vi "Add User.vi"(8 "error in":errorcluster, 9 "Path":path) -> (0 "error out":errorcluster)   [LabVIEW 2015]
uses:
  <vilib>/Utility/file.llb/Read Delimited Spreadsheet (string).vi
  <vilib>/Utility/file.llb/Write Delimited Spreadsheet (string).vi
panel:
  in  "hide(F)/show(T)":bool
  in  "Cancel":bool
  in  "OK":bool
  in  "User Name":string
  in  "Password":string
  in  "Designation":u16(ring) items=["Select the Designation", "Operator", "Supevisor", "Admin"]
  # "Add User Credential"
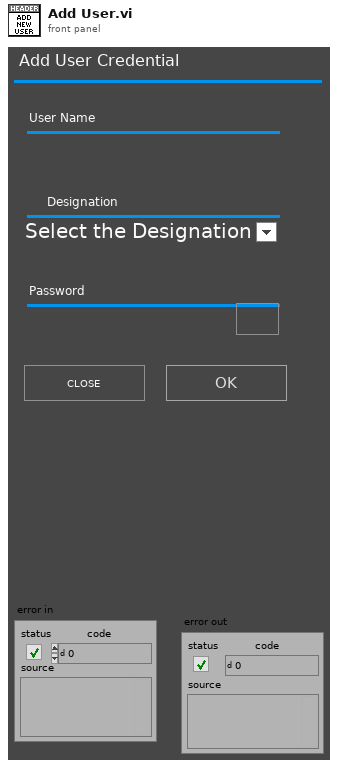
[diagram p1: front panel]
types:
  T1 = enum8{"Enabled", "Disabled", "Disabled and Grayed Out"}
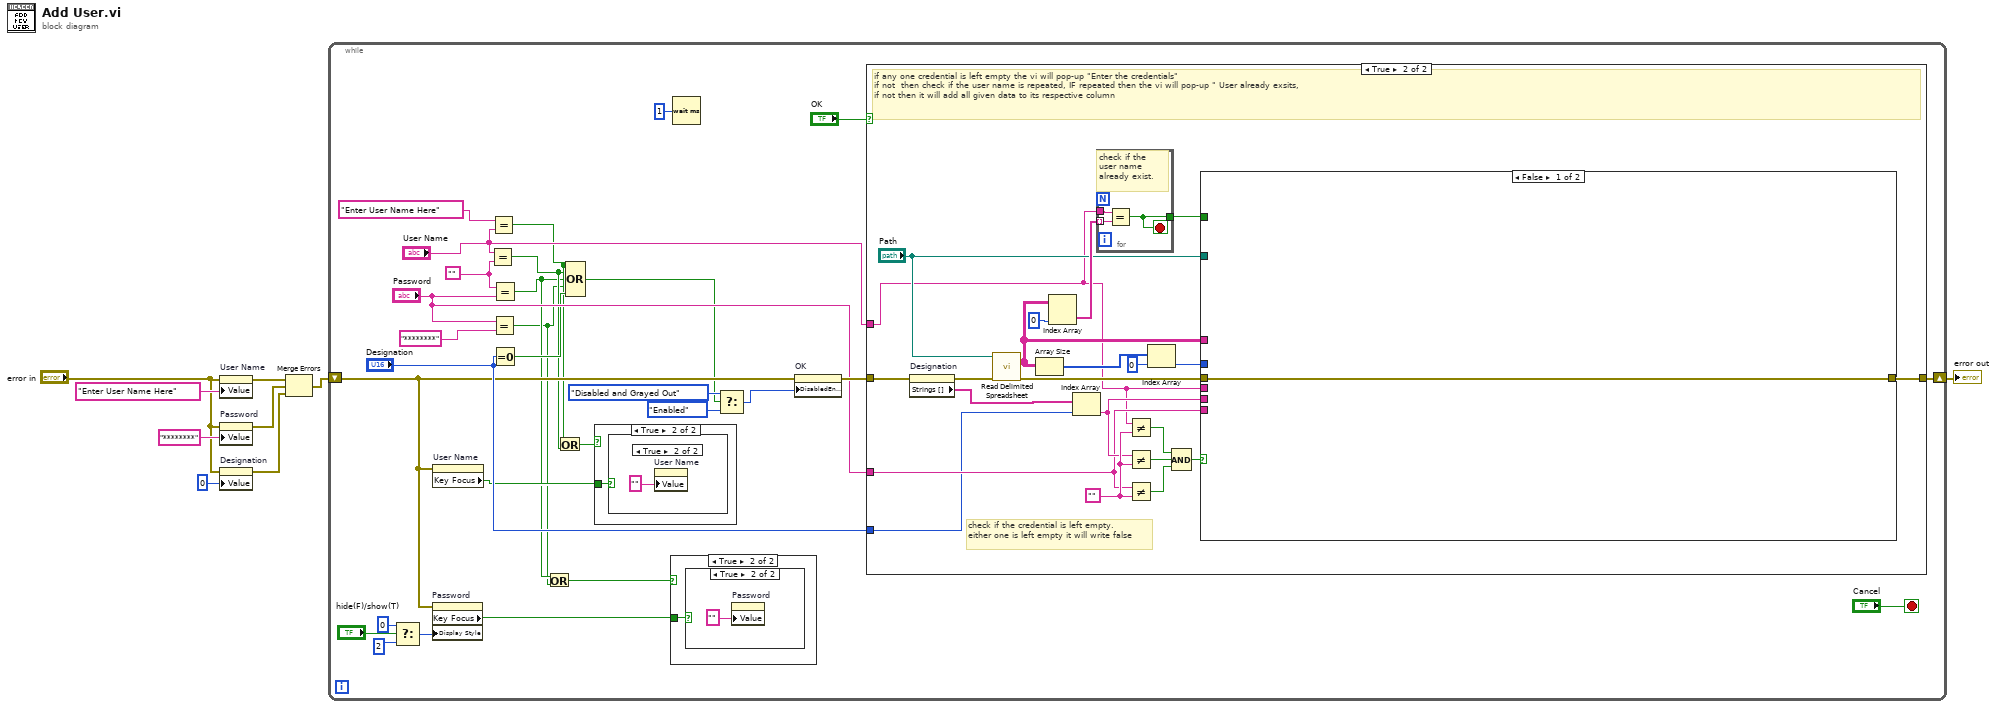
[diagram p0: block diagram]
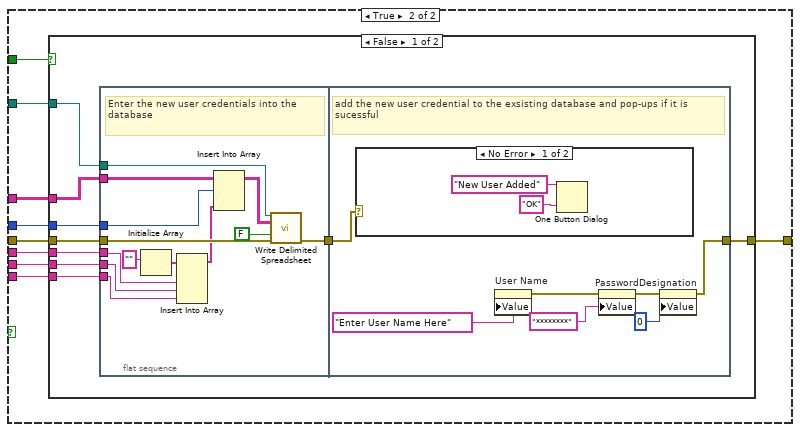
[diagram p7: hidden frame]
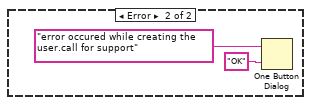
[diagram p8: hidden frame]
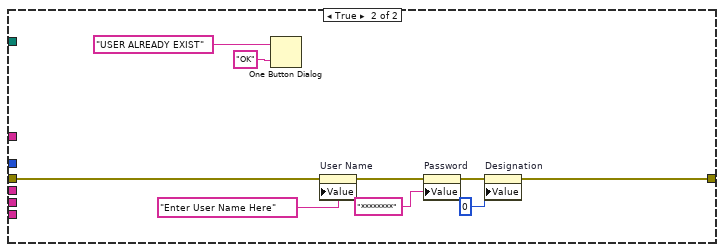
[diagram p9: hidden frame]
diagram:
  n1 = property on="User Name" class="Str"(error in="error in", "Value"="Enter User Name Here") -> (error out=w3:errorcluster)  [unwired: 1 in, 1 out]
  n2 = property on="Password" class="Str"(error in="error in", "Value"="********") -> (error out=w4:errorcluster)  [unwired: 1 in, 1 out]
  n3 = property on="Designation" class="Ring (strict)"(error in="error in", "Value"=0) -> (error out=w5:errorcluster)  [unwired: 1 in, 1 out]
  n4 = Merge Errors(w3, w4, w5) -> (w1:errorcluster)
  n5 = while {
    shift-right: [w36] -> w9
    shift-left: w1 -> [w24]
    stop <- "Cancel" stop-if-true
    w34 = ""
    n6 = Select(t=u32 0, s="hide(F)/show(T)", f=u32 2 ("Display Style")) -> (s? t:f=w11:u32)
    n7 = property on="Password" class="Str"(error in=w24, "Display Style"=w11) -> ("Key Focus"=w12:bool)  [unwired: 1 in, 2 out]
    n8 = property on="User Name" class="Str"(error in=w24) -> ("Key Focus"=w16:bool)  [unwired: 1 in, 2 out]
    n9 = Equal?(x="User Name", y=w34) -> (x = y?=w18:bool)
    n10 = Equal?(x="Enter User Name Here", y="User Name") -> (x = y?=w19:bool)
    n11 = Equal?(x="Password", y="********") -> (x = y?=w13:bool)
    n12 = Equal?(x=w34, y="Password") -> (x = y?=w14:bool)
    n13 = Equal To 0?(x="Designation") -> (x = 0?=w28:bool)
    n14 = Or(x=w14, y=w13) -> (x .or. y?=w15:bool)
    n15 = Or(x=w19, y=w18) -> (x .or. y?=w17:bool)
    n16 = Compound Arithmetic op=OR(w19, w18, w14, w13, w28) -> (w22:bool)
    n17 = case shown="True" w17 {
      tunnel: w16 -> [_ w41]
      frame False {
      }
      frame True {
        n18 = case shown="True" w41 {
          frame False {
          }
          frame True {
            n19 = property on="User Name" class="Str"("Value"="" ("User Name")) -> ()  [unwired: 2 in, 2 out]
          }
        }
      }
    }
    n20 = case shown="True" w15 {
      tunnel: w12 -> [_ w39]
      frame False {
      }
      frame True {
        n21 = case shown="True" w39 {
          frame False {
          }
          frame True {
            n22 = property on="Password" class="Str"("Value"="" ("User Name")) -> ()  [unwired: 2 in, 2 out]
          }
        }
      }
    }
    n23 = Wait (ms)(milliseconds to wait=u32 1) -> ()  [unwired: 1 out]
    n24 = Select(t=T1."Disabled and Grayed Out" ("Disabled"), s=w22, f=T1."Enabled") -> (s? t:f=w20:T1)
    n25 = property on="OK" class="Bool"(error in=w24, "DisabledEnum"=w20) -> (error out=w35:errorcluster)  [unwired: 1 in, 1 out]
    n26 = case shown="True" "OK" {
      tunnel: w35 -> [w43 w46]
      tunnel: [w43 w50] -> w36
      tunnel: "User Name" -> [_ w48]
      tunnel: "Password" -> [_ w49]
      tunnel: "Designation" -> [_ w47]
      frame False {
      }
      frame True {
        w63 = ""
        # "check if the credential is left empty. either one is left empty it will write false"
        # "if any one credential is left empty the vi will pop-up \"Enter the credentials\" \nif not  then check if the user name is repeated, IF repeated then the vi will pop-up \" User already exsits,\nif not then it will add all given data to its respective column"
        n27 = property on="Designation" class="Ring (strict)"(error in=w46) -> (error out=w45:errorcluster, "Strings []"=w44:string[])  [unwired: 1 in, 1 out]
        n28 = call-poly <vilib>:"Read Delimited Spreadsheet.vi"("file path (dialog if empty)"="Path", "error in (no error)"=w45) -> ("all rows"=w52:string[][], "error out"=w51:errorcluster)  [unwired: 8 in, 4 out]
        n29 = Array Size(array=w52) -> (size(s)=w65:i32[])
        n30 = Index Array(array=w52, index (col)=0 ("disabled index (col)")) -> (element=w57:string[])  [unwired: 1 in]
        n31 = Index Array(array=w44, index=w47) -> (element=w53:string)
        n32 = for {
          tunnel: [w66] -> w58
          tunnel: w57 -> [w68] mode=indexing
          tunnel: w48 -> [w67]
          stop <- w66 stop-if-true
          # "check if the user name\nalready exist."
          n33 = Equal?(x=w67, y=w68) -> (x = y?=w66:bool)
        }
        n34 = Not Equal?(x=w48, y=w63) -> (x != y?=w62:bool)
        n35 = Not Equal?(x=w53, y=w63) -> (x != y?=w61:bool)
        n36 = Not Equal?(x=w49, y=w63) -> (x != y?=w60:bool)
        n37 = Index Array(array=w65, index=0) -> (element=w56:i32)
        n38 = Compound Arithmetic op=AND(w62, w61, w60) -> (w55:bool)
        n39 = case shown="False" w55 {
          tunnel: w58 -> [_ w78]
          tunnel: w52 -> [_ w77]
          tunnel: w56 -> [_ w76]
          tunnel: "Path" -> [_ w75]
          tunnel: w49 -> [_ w74]
          tunnel: w53 -> [_ w73]
          tunnel: w48 -> [_ w72]
          tunnel: w51 -> [w69 w71]
          tunnel: [w69 w70] -> w50
          frame False {
          }
          frame True {
            n40 = case shown="False" w78 {
              tunnel: w77 -> [w87 _]
              tunnel: w76 -> [w82 _]
              tunnel: w75 -> [w86 _]
              tunnel: w74 -> [w85 _]
              tunnel: w73 -> [w84 _]
              tunnel: w72 -> [w83 _]
              tunnel: w71 -> [w80 w113]
              tunnel: [w79 w112] -> w70
              frame False {
                n41 = flat-sequence {
                  tunnel: w87 -> [w99]
                  tunnel: w86 -> [w97]
                  tunnel: w85 -> [w89]
                  tunnel: w84 -> [w90]
                  tunnel: w83 -> [w91]
                  tunnel: w82 -> [w96]
                  tunnel: [w95] -> w81
                  tunnel: w80 -> [w94]
                  tunnel: w81 -> [w102]
                  tunnel: [w101] -> w79
                  frame #0 {
                    # "Enter the new user credentials into the database"
                    n42 = Initialize Array("") -> (w92:string[])  [unwired: 1 in]
                    n43 = Insert Into Array(array=w92, new element #1=w91, new element #2=w90, new element #3=w89) -> (w88:string[])  [unwired: 1 in]
                    n44 = Insert Into Array(array=w99, index (row)=w96, new element=w88) -> (w98:string[][])  [unwired: 1 in]
                    n45 = call-poly <vilib>:"Write Delimited Spreadsheet.vi"("file path (dialog if empty)"=w97, "2D data"=w98, "append to file? (F)"=FALSE, "error in (no error)"=w94) -> ("error out"=w95:errorcluster)  [unwired: 10 in, 1 out]
                  }
                  frame #1 {
                    # "add the new user credential to the exsisting database and pop-ups if it is sucessful"
                    n46 = case shown="No Error" w102 {
                      frame No Error {
                        n47 = One Button Dialog(message="New User Added", button name ("OK")="OK") -> ()  [unwired: 1 out]
                      }
                      frame Error {
                        n48 = One Button Dialog(message="error occured while creating the user.call for support", button name ("OK")="OK") -> ()  [unwired: 1 out]
                      }
                    }
                    n49 = property on="User Name" class="Str"("Value"="Enter User Name Here") -> (error out=w104:errorcluster)  [unwired: 2 in, 1 out]
                    n50 = property on="Password" class="Str"(error in=w104, "Value"="********") -> (error out=w103:errorcluster)  [unwired: 1 in, 1 out]
                    n51 = property on="Designation" class="Ring (strict)"(error in=w103, "Value"=0) -> (error out=w101:errorcluster)  [unwired: 1 in, 1 out]
                  }
                }
              }
              frame True {
                n52 = One Button Dialog(message="USER ALREADY EXIST", button name ("OK")="OK") -> ()  [unwired: 1 out]
                n53 = property on="User Name" class="Str"(error in=w113, "Value"="Enter User Name Here") -> (error out=w115:errorcluster)  [unwired: 1 in, 1 out]
                n54 = property on="Password" class="Str"(error in=w115, "Value"="********") -> (error out=w114:errorcluster)  [unwired: 1 in, 1 out]
                n55 = property on="Designation" class="Ring (strict)"(error in=w114, "Value"=0) -> (error out=w112:errorcluster)  [unwired: 1 in, 1 out]
              }
            }
          }
        }
      }
    }
  }
  "error out" <- w9
